vi "Set Thermocouple Meas Mode.vi"(8 "error in (no error)":errorcluster, 10 "Temperature Units (22: Temperature in degrees Celsius)":u32(ring)=22 items=["Unitless", "Frequency in units of hertz", "Frequency in units of kilohertz", "Frequency in units of megahertz", "Volts in units of microvolts", "Volts in units of millivolts", "Volts in units of volts", "Volts in units of kilovolts", "Current in units of microamperes", "Current in units of milliamps", "Current in units of amps", "Percent", "Parts-per-million", "Volts in units of decibels referenced to 1 milliwatt into 600 W load", "Resistance in units of ohms", "Resistance in units of kilohms", "Resistance in units of megohms", "Capacitance in units of nanofarads", "Capacitance in units of picofarads", "Capacitance in units of  microfarads", "Capacitance in units of millifarads", "Capacitance in units of farads", "Temperature in degrees Celsius", "Temperature in degrees Fahrenheit", "Period in units of nanoseconds", "Period in units of microseconds", "Period in units of milliseconds", "Period in units of seconds", "Pound-force pre square inch", "Meters of mercury", "Inches of mercury", "Inches of water", "Feet of water", "Meters of water", "Bar", "Pascal", "Grams per centimeter squared", "Inches of water @ 60 degrees Farhenheit", "Decibels"], 11 "VISA resource name":refnum<visa-resource-name>) -> (0 "error out":errorcluster, 3 "VISA resource name out":refnum<visa-resource-name>)   [LabVIEW 2011, in "Fluke 5XXX Series Multicalibrators.lvlib"]
doc: "This VI selects mode to measure the thermocouple temperature that is attached to the Calibrator TC terminals.\n\nNote:\n\nThis VI is available only for instrument models 5500A and 5520A."
uses:
  Fluke 5XXX Series Multicalibrators.lvlib
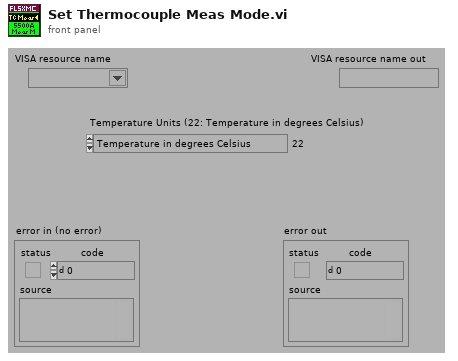
[diagram p1: front panel]
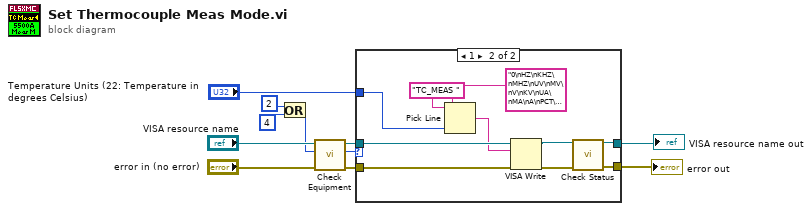
[diagram p0: block diagram]
diagram:
  n1 = Or(x=2 ("Numeric"), y=4 ("Numeric")) -> (x .or. y?=w2:i32)
  n2 = call "Check Equipment.vi"("error in (no error)"="error in (no error)", "Bit Mask"=w2, "VISA resource name"="VISA resource name") -> ("error out"=w11:errorcluster, "Present?"=w10:u32, "VISA resource name out"=w9:refnum<visa-resource-name>)  [unwired: 6 in]
  n3 = case shown="1" w10 {
    tunnel: [w12 w16] -> w5
    tunnel: w11 -> [w13 w22]
    tunnel: w9 -> [w12 w21]
    tunnel: [w13 w19] -> w6
    tunnel: "Temperature Units (22: Temperature in degrees Celsius)" -> [_ w15]
    frame 0, Default {
    }
    frame 1 {
      n4 = Pick Line(string ("")="TC_MEAS " ("Reset Command"), multi-line string="0\nHZ\nKHZ\nMHZ\nUV\nMV\nV\nKV\nUA\nMA\nA\nPCT\nPPM\nDBM\nOHM\nKOHM\nMOHM\nNF\nPF\nUF\nMF\nF\nCEL\nFAR\nNS\nUS\nMS\nS\nPSI\nMHG\nINHG\nINH2O\nFTH2O\nMH2O\nBAR\nPAL\nG/CM2\nINH2O60F\nDB", line index=w15) -> (output string=w20:string)
      n5 = VISA Write(VISA resource name=w21, write buffer=w20, error in (no error)=w22) -> (VISA resource name out=w17:refnum<visa-resource-name>, error out=w18:errorcluster)  [unwired: 1 out]
      n6 = call "Check Status.vi"("VISA resource name"=w17, "error in (no error)"=w18) -> ("VISA resource name out"=w16:refnum<visa-resource-name>, "error out"=w19:errorcluster)  [unwired: 12 in]
    }
  }
  "VISA resource name out" <- w5
  "error out" <- w6
